vi "Write Filter.vi"(8 "error in (no error)":errorcluster, 10 "Filter":T1[](array[typedef]) {"IPV4 Filter"."Protocol" items=["ICMP"=1, "IGMP"=2, "TCP"=6, "UDP"=17]; "IPV4 Filter"."Dest IP Address" format="%.0x"; "IPV4 Filter"."Source IP Address" format="%.0x"; "L2 Filter"."EtherType" format="%04x"; "L2 Filter"."SMAC" format="%02x"; "L2 Filter"."DMAC" format="%02x"}, 11 "CAN_RW_CORE in":refnum<class "L2ENET_RW_CORE.lvclass">) -> (0 "error out":errorcluster, 3 "CAN_RW_CORE out":refnum<class "L2ENET_RW_CORE.lvclass">)   [LabVIEW 2021, in "L2ENET_RW_CORE.lvclass"]
uses:
  L2ENET_RW_CORE.lvclass
  L2ENET_RW_CORE.lvclass/L2ENET_RW_CORE.ctl
  <vilib>/CIF Foundation/CIF Enet Parse and Build/typedef/L2 & L3/L2 Filter.ctl
  <vilib>/CIF Foundation/CIF Enet Parse and Build/Ethernet_Parse_Build_CIF.lvlib
  <vilib>/CIF Foundation/CIF Enet Parse and Build/typedef/L2 & L3/IPV4 Protocol Ring.ctl
  <vilib>/CIF Foundation/CIF Enet Parse and Build/typedef/L2 & L3/IPV4 Filter.ctl
  <vilib>/CIF Foundation/CIF Enet Parse and Build/typedef/L2 & L3/Filter.ctl
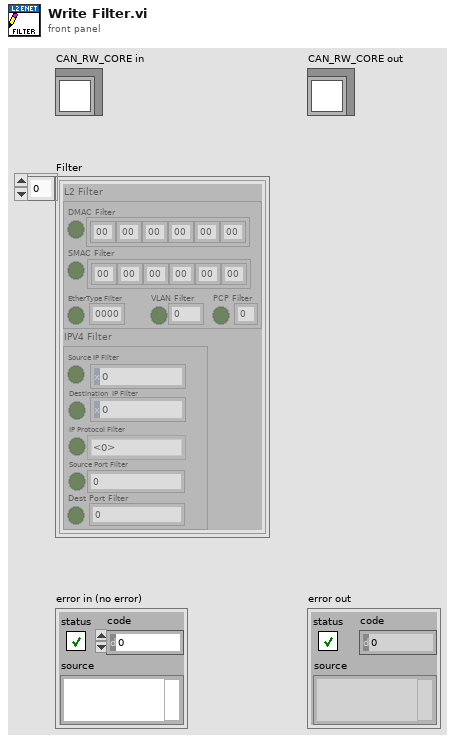
[diagram p1: front panel]
types:
  T1 = typedef "Ethernet_Parse_Build_CIF.lvlib/Filter.ctl" = cluster{"L2 Filter":T2, "IPV4 Filter":T3}
  T2 = typedef "Ethernet_Parse_Build_CIF.lvlib/L2 Filter.ctl" = cluster{"DMAC Filter":bool, "DMAC":u8[], "SMAC Filter":bool, "SMAC":u8[], "EtherType Filter":bool, "EtherType":u16, "VLAN Filter":bool, "VLAN":u16, "PCP Filter":bool, "PCP":u8}
  T3 = typedef "Ethernet_Parse_Build_CIF.lvlib/IPV4 Filter.ctl" = cluster{"Source IP Filter":bool, "Source IP Address":u32, "Destination  IP Filter":bool, "Dest IP Address":u32, "IP Protocol Filter":bool, "Protocol":T4, "Source Port Filter":bool, "Source Port":u16, "Dest Port Filter ":bool, "Dest Port":u16}
  T4 = typedef "Ethernet_Parse_Build_CIF.lvlib/IPV4 Protocol Ring.ctl" = u8
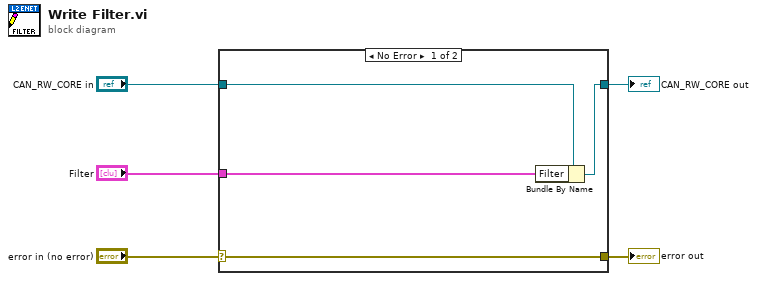
[diagram p0: block diagram]
diagram:
  n1 = case shown="No Error" "error in (no error)" {
    selector: "error in (no error)" -> [w9 w10]
    tunnel: [w9 w10] -> w4
    tunnel: [w7 w11] -> w2
    tunnel: "CAN_RW_CORE in" -> [w8 w11]
    tunnel: "Filter" -> [w6 _]
    frame No Error {
      n2 = Bundle By Name(cluster=w8, "Filter"=w6) -> (w7:refnum<class "L2ENET_RW_CORE.lvclass">)
    }
    frame Error {
    }
  }
  "error out" <- w4
  "CAN_RW_CORE out" <- w2
